vi "Machmodul Spannung zu Temp (SubVI).vi"(2 "Temp PT 100 soll":dbl, 3 "U ist":fxp<+/-,16,4>) -> (0 "U soll":fxp<+/-,16,4> format="%.14g", 1 "Temp PT 100 ist":dbl)   [LabVIEW 2010]
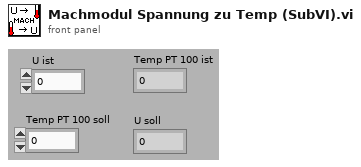
[diagram p1: front panel]
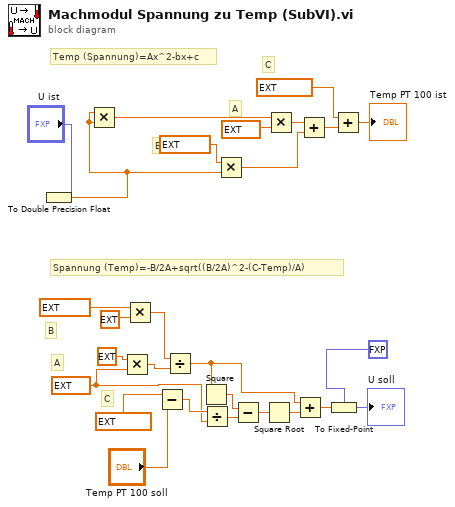
[diagram p0: block diagram]
diagram:
  w7 = ext 6.0782 ("y")
  # "C"
  # "A"
  # "B"
  # "Spannung (Temp)=-B/2A+sqrt((B/2A)^2-(C-Temp)/A)"
  # "Temp (Spannung)=Ax^2-bx+c"
  # "C"
  # "A"
  # "B"
  n1 = To Double Precision Float(number="U ist") -> (double precision float=w3:dbl)
  n2 = Multiply(x=w3, y=w3) -> (x*y=w27:dbl)
  n3 = Multiply(x=ext 2.0 ("y"), y=w7) -> (x*y=w15:ext)
  n4 = Multiply(x=ext 153.16209999999999999 ("y"), y=ext -1.0) -> (x*y=w17:ext)
  n5 = Subtract(x=ext -237.2852 ("y"), y="Temp PT 100 soll") -> (x-y=w12:ext)
  n6 = Divide(x=w17, y=w15) -> (x/y=w9:ext)
  n7 = Square(x=w9) -> (x^2=w14:ext)
  n8 = Divide(x=w12, y=w7) -> (x/y=w11:ext)
  n9 = Multiply(x=ext 153.16209999999999999 ("y"), y=w3) -> (x*y=w24:ext)
  n10 = Subtract(x=w14, y=w11) -> (x-y=w10:ext)
  n11 = Square Root(x=w10) -> (sqrt(x)=w8:ext)
  n12 = Multiply(x=w27, y=ext 6.0782) -> (x*y=w23:ext)
  n13 = Add(x=w9, y=w8) -> (x+y=w6:ext)
  n14 = Add(x=w23, y=w24) -> (x+y=w22:ext)
  n15 = To Fixed-Point(fixed-point type=fxp<+/-,16,4> 0.0 ("Festkommatyp"), number=w6) -> (fixed-point=→"U soll":fxp<+/-,16,4>)
  n16 = Add(x=ext -237.2852 ("y"), y=w22) -> (x+y=→"Temp PT 100 ist":ext)
